vi "SR SIM921 Get Active Curve.vi"(4 "Error In":errorcluster, 6 "SIM Slot #":T1(radio), 7 "VISA session":refnum<visa-resource-name>) -> (0 "Error Out":errorcluster, 2 "Curve #":i32, 3 "dup VISA session":refnum<visa-resource-name>)   [LabVIEW 2020]
doc: "This VI reads a curve header from the LakeShore Model 370 AC Resistance Bridge and returns the parsed data.\nScott Hannahs, <sth@magnet.fsu.edu> NHMFL-FSU, May 2003"
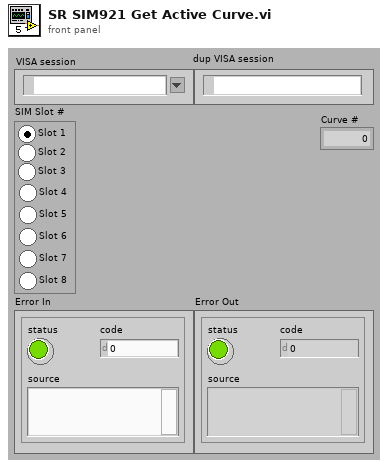
[diagram p1: front panel]
types:
  T1 = enum32{"Slot 1", "Slot 2", "Slot 3", "Slot 4", "Slot 5", "Slot 6", "Slot 7", "Slot 8"}
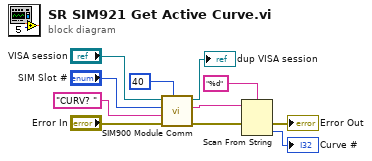
[diagram p0: block diagram]
diagram:
  n1 = call "SIM900 Module Comm.vi"("Wait (ms)"=u32 40 ("wait (mS)"), "Error In"="Error In", "Query"="CURV? " ("String to Write"), "Slot"="SIM Slot #", "VISA Resource Name"="VISA session") -> ("Error Out"=w4:errorcluster, "Response"=w11:string, "dup VISA Session"=→"dup VISA session":refnum<visa-resource-name>)  [unwired: 4 in]
  n2 = Scan From String(format string="%d", input string=w11, error in=w4) -> (error out=→"Error Out":errorcluster, output 1=→"Curve #":i32)  [unwired: 2 in, 2 out]
